vi "Renew Blob Lease.vi"(6 "Lease ID":string, 8 "error in (no error)":errorcluster, 9 "Blob":string, 10 "Container":string, 11 "Azure Session in":refnum<class "Session.lvclass">) -> (0 "error out":errorcluster, 3 "Azure Session out":refnum<class "Session.lvclass">)   [LabVIEW 2015, in "NI_Azure_Blob.lvlib"]
doc: "Renew an existing lease on a blob."
uses:
  NI_Azure_Blob.lvlib
  Core/Session/Session.lvclass
  Core/Name Value Pair.ctl
  Lease Action.ctl
  Core/Session/Session.lvclass/Session.ctl
  Core/Session/Write Request Headers.vi
  Core/Session/Write Request Parameters.vi
  Core/Session/Write HTTP Verb.vi
  Core/Session/Write URL Suffix.vi
  Core/NI_Azure_Core.lvlib
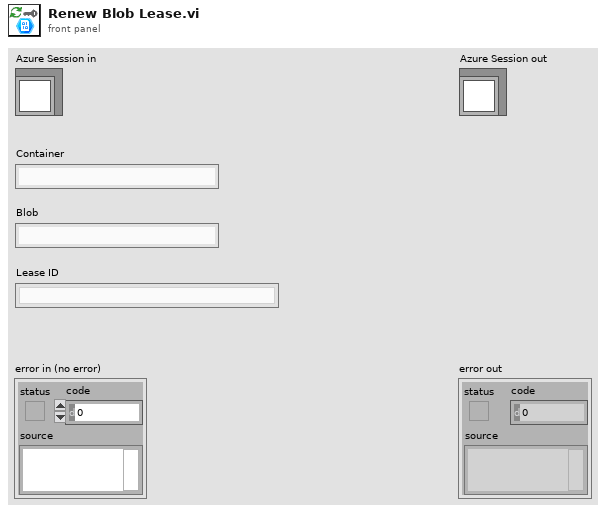
[diagram p1: front panel]
types:
  T1 = typedef "NI_Azure_Blob.lvlib/Lease Action.ctl" = enum16{"acquire", "renew", "change", "release", "break"}
  T2 = typedef "NI_Azure_Core.lvlib/Name Value Pair.ctl" = cluster{"name":string, "value":string}
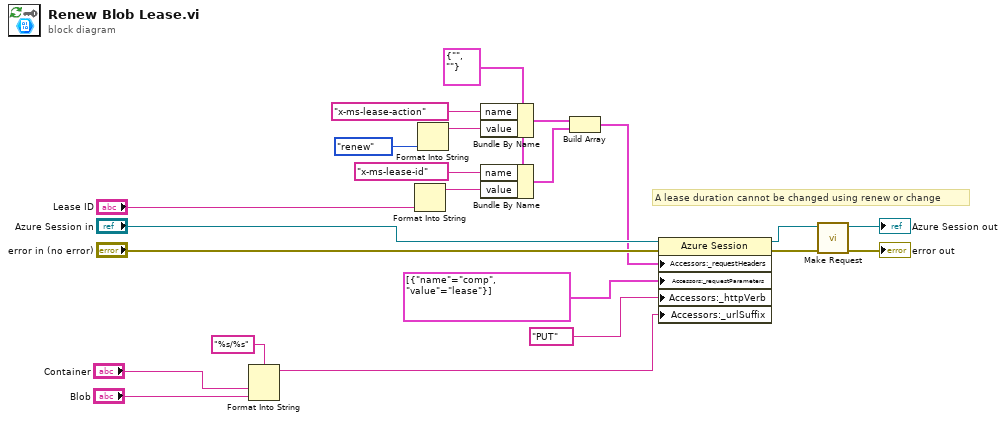
[diagram p0: block diagram]
diagram:
  w13 = T2 {"name"="", "value"=""} ("Cluster")
  # "A lease duration cannot be changed using renew or change"
  n1 = Format Into String(format string="%s/%s", "Container", "Blob") -> (resulting string=w1:string)  [unwired: 2 in, 1 out]
  n2 = Format Into String("Lease ID") -> (resulting string=w11:string)  [unwired: 3 in, 1 out]
  n3 = Format Into String(Lease_Action."renew" ("Lease action")) -> (resulting string=w15:string)  [unwired: 3 in, 1 out]
  n4 = Bundle By Name(cluster=w13, "name"="x-ms-lease-action" ("header"), "value"=w15) -> (w17:T2)
  n5 = Bundle By Name(cluster=w13, "name"="x-ms-lease-id" ("header"), "value"=w11) -> (w10:T2)
  n6 = Build Array(w17, w10) -> (w3:T2[])
  n7 = property class="Azure Session"(reference="Azure Session in", error in="error in (no error)", "Accessors:_requestHeaders"=w3, "Accessors:_requestParameters"=T2[] [{"name"="comp", "value"="lease"}] ("request parameters"), "Accessors:_httpVerb"="PUT" ("HTTP-Verb"), "Accessors:_urlSuffix"=w1) -> (reference out=w5:refnum<class "Session.lvclass">, error out=w7:errorcluster)
  n8 = call "Make Request.vi"("error in (no error)"=w7, "Session in"=w5) -> ("error out"=→"error out":errorcluster, "Session out"=→"Azure Session out":refnum<class "Session.lvclass">)  [unwired: 7 in, 1 out]
